vi "FGV - Initialization Status.vi"(7 "Status":enum16{"Uninitialized", "Initialized"}(ring), 8 "error in (no error)":errorcluster, 11 "Actions":T1=enum."Clear") -> (0 "error out":errorcluster, 3 "Status out":enum16{"Uninitialized", "Initialized"}(ring))   [LabVIEW 2017]
uses:
  Controls/FGV Actions.ctl
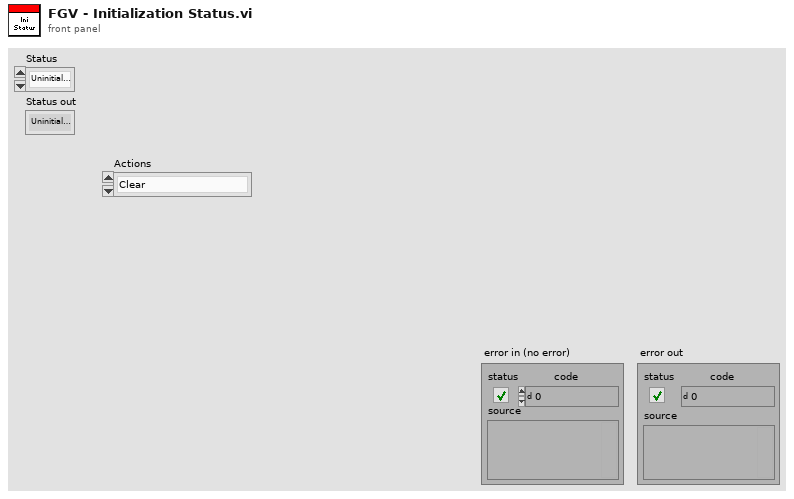
[diagram p1: front panel]
types:
  T1 = typedef "FGV Actions.ctl" = enum16{"Init", "Set", "Get", "Clear"}
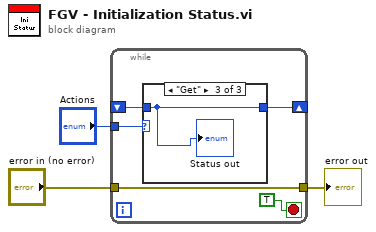
[diagram p0: block diagram]
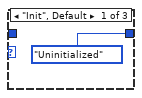
[diagram p2: hidden frame]
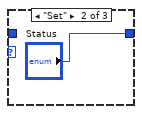
[diagram p3: hidden frame]
diagram:
  n1 = while {
    tunnel: "Actions" -> [w8]
    shift-right: [w6] -> _
    shift-left: _ -> [w5]
    tunnel: "error in (no error)" -> [w4]
    tunnel: [w4] -> w1
    stop <- TRUE stop-if-true
    n2 = case shown="\"Get\"" w8 {
      tunnel: [enum16{"Uninitialized", "Initialized"}."Uninitialized" "Status" w11] -> w6
      tunnel: w5 -> [_ _ w11]
      frame "Init", Default {
      }
      frame "Set" {
      }
      frame "Get" {
        "Status out" <- w11
      }
    }
  }
  "error out" <- w1
